vi "FPGA_R_ADC_loadcell_W_DAC.vi"() -> ()   [LabVIEW 2018]
uses:
  <vilib>/rvi/Emulation/niFpgaGetClockAttributes.vi
  <vilib>/rvi/Emulation/niFpgaSctlEmulationGetInTimedLoop.vi
  <vilib>/rvi/Emulation/niFpgaEmulationReportErrorSimple.vi
  <vilib>/rvi/eio/common/nirviEmuTemplateMethod_errors.vi
  <vilib>/rvi/Emulation/niFpgaCriticalErrorInLSC.vi
  <vilib>/eio/EIONode/EIONode.xnode
panel:
  out "Data array":bool[](array[boolean])
  in  "stop":bool
  in  "DAC 3 write":bool[](array[boolean])=[FALSE, FALSE, FALSE, FALSE, FALSE, FALSE, FALSE, FALSE, FALSE, FALSE, FALSE, FALSE, FALSE, FALSE, FALSE, FALSE]
  in  "DAC 2 write":bool[](array[boolean])=[FALSE, FALSE, FALSE, FALSE, FALSE, FALSE, FALSE, FALSE, FALSE, FALSE, FALSE, FALSE, FALSE, FALSE, FALSE, FALSE]
  in  "DAC 1 write":bool[](array[boolean])=[FALSE, FALSE, FALSE, FALSE, FALSE, FALSE, FALSE, FALSE, FALSE, FALSE, FALSE, FALSE, FALSE, FALSE, FALSE, FALSE]
  out "ADC read":bool[](array[boolean])
  in  "ADC write":bool[](array[boolean])=[FALSE, FALSE, FALSE, FALSE, FALSE, TRUE, FALSE, FALSE, FALSE, FALSE, FALSE, FALSE, FALSE, FALSE, FALSE, FALSE]
  in  "Stop":bool
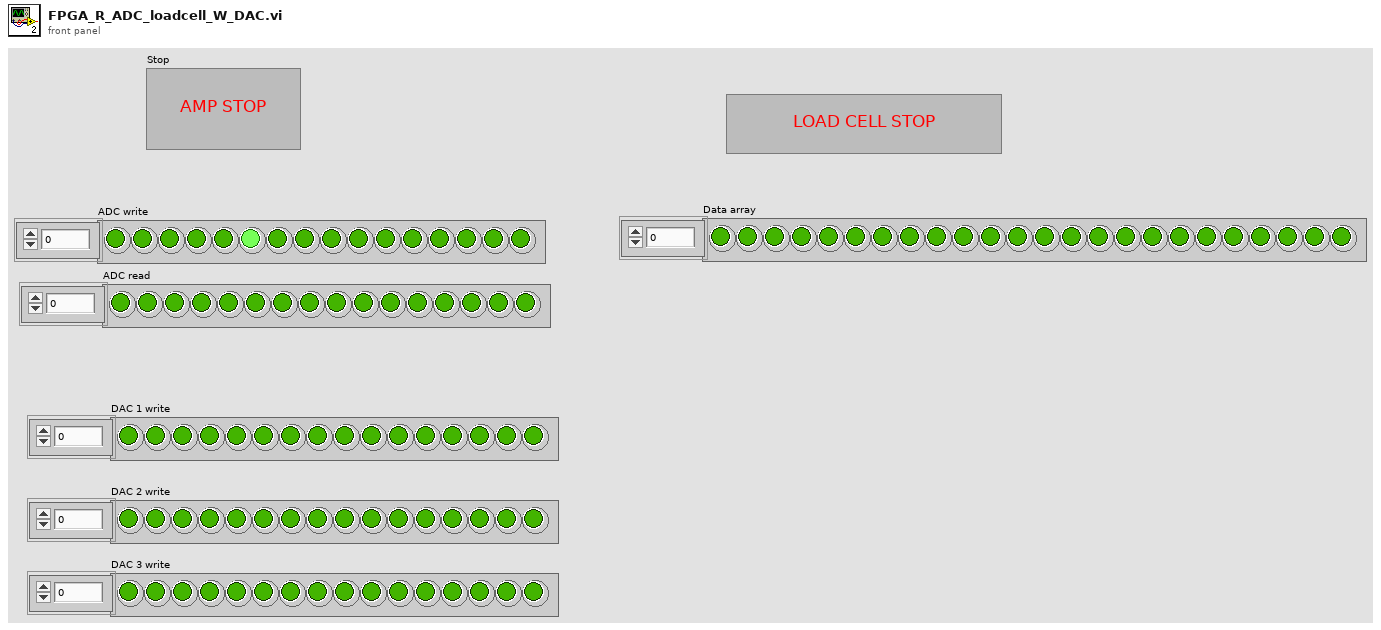
[diagram p1: front panel]
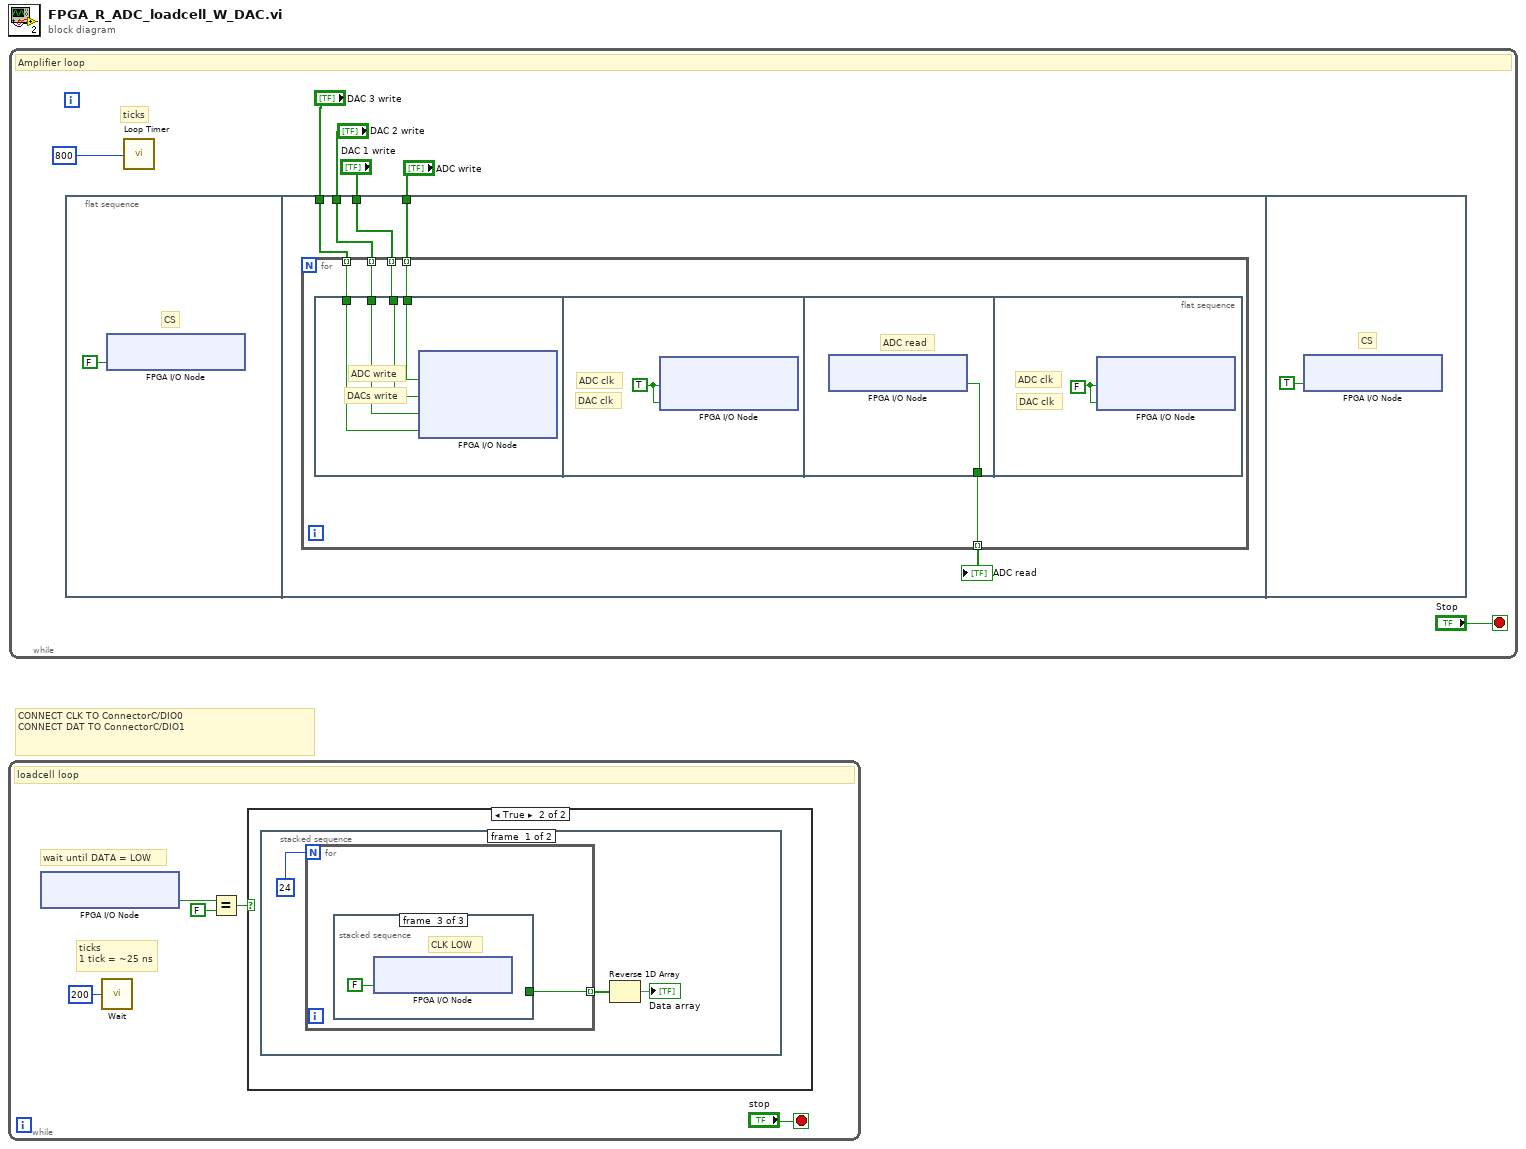
[diagram p0: block diagram]
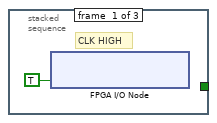
[diagram p3: hidden frame]
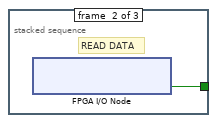
[diagram p4: hidden frame]
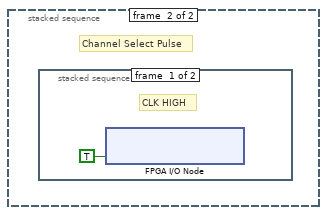
[diagram p5: hidden frame]
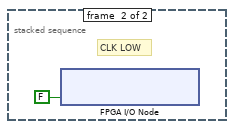
[diagram p6: hidden frame]
diagram:
  # "CONNECT CLK TO ConnectorC/DIO0\nCONNECT DAT TO ConnectorC/DIO1"
  n1 = while {
    stop <- "stop" stop-if-true
    # "ticks\n1 tick = ~25 ns"
    # "wait until DATA = LOW"
    # "loadcell loop"
    n2 = xnode "FPGA I/O Node"() -> ("ConnectorC/DIO1"=w4:bool)  [unwired: 1 in, 1 out]
    n3 = call "Wait"("Count(Ticks)"=u32 200) -> ()  [unwired: 1 out]
    n4 = Equal?(x=w4, y=FALSE) -> (x = y?=w2:bool)
    n5 = case shown="True" w2 {
      frame False {
      }
      frame True {
        n6 = stacked-sequence {
          frame #0 {
            n7 = for {
              N: 24 -> [_]
              tunnel: [w9] -> w7 mode=indexing
              n8 = stacked-sequence {
                tunnel: [_ w11 _] -> w9
                frame #0 {
                  # "CLK HIGH"
                  n9 = xnode "FPGA I/O Node"("ConnectorC/DIO0"=TRUE ("ConnectorB/DIO0")) -> ()  [unwired: 1 in, 1 out]
                }
                frame #1 {
                  # "READ DATA"
                  n10 = xnode "FPGA I/O Node"() -> ("ConnectorC/DIO1"=w11:bool)  [unwired: 1 in, 1 out]
                }
                frame #2 {
                  # "CLK LOW"
                  n11 = xnode "FPGA I/O Node"("ConnectorC/DIO0"=FALSE ("ConnectorB/DIO0")) -> ()  [unwired: 1 in, 1 out]
                }
              }
            }
            n12 = Reverse 1D Array(array=w7) -> (reversed array=→"Data array":bool[])
          }
          frame #1 {
            # "Channel Select Pulse"
            n13 = stacked-sequence {
              frame #0 {
                # "CLK HIGH"
                n14 = xnode "FPGA I/O Node"("ConnectorC/DIO0"=TRUE ("ConnectorB/DIO0")) -> ()  [unwired: 1 in, 1 out]
              }
              frame #1 {
                # "CLK LOW"
                n15 = xnode "FPGA I/O Node"("ConnectorC/DIO0"=FALSE ("ConnectorB/DIO0")) -> ()  [unwired: 1 in, 1 out]
              }
            }
          }
        }
      }
    }
  }
  n16 = while {
    stop <- "Stop" stop-if-true
    # "ticks"
    # "Amplifier loop"
    n17 = flat-sequence {
      tunnel: "ADC write" -> [w26]
      tunnel: "DAC 1 write" -> [w24]
      tunnel: "DAC 2 write" -> [w23]
      tunnel: "DAC 3 write" -> [w22]
      frame #0 {
        # "CS"
        n18 = xnode "FPGA I/O Node"("ConnectorA/DIO4"=FALSE) -> ()  [unwired: 1 in, 1 out]
      }
      frame #1 {
        n19 = for {
          tunnel: w26 -> [w31] mode=indexing
          tunnel: [w30] -> w25 mode=indexing
          tunnel: w24 -> [w29] mode=indexing
          tunnel: w23 -> [w28] mode=indexing
          tunnel: w22 -> [w27] mode=indexing
          n20 = flat-sequence {
            tunnel: w31 -> [w35]
            tunnel: w29 -> [w34]
            tunnel: w28 -> [w33]
            tunnel: w27 -> [w32]
            tunnel: [w37] -> w30
            frame #0 {
              # "DACs write"
              # "ADC write"
              n21 = xnode "FPGA I/O Node"("ConnectorA/DIO2"=w35, "ConnectorA/DIO6"=w34, "ConnectorA/DIO7"=w33, "ConnectorA/DIO8"=w32) -> ()  [unwired: 4 in, 4 out]
            }
            frame #1 {
              w36 = TRUE ("ConnectorA/DIO3")
              # "DAC clk"
              # "ADC clk"
              n22 = xnode "FPGA I/O Node"("ConnectorA/DIO3"=w36, "ConnectorA/DIO5"=w36) -> ()  [unwired: 2 in, 2 out]
            }
            frame #2 {
              # "ADC read"
              n23 = xnode "FPGA I/O Node"() -> ("ConnectorA/DIO1"=w37:bool)  [unwired: 1 in, 1 out]
            }
            frame #3 {
              w38 = FALSE ("ConnectorA/DIO3")
              # "DAC clk"
              # "ADC clk"
              n24 = xnode "FPGA I/O Node"("ConnectorA/DIO3"=w38, "ConnectorA/DIO5"=w38) -> ()  [unwired: 2 in, 2 out]
            }
          }
        }
        "ADC read" <- w25
      }
      frame #2 {
        # "CS"
        n25 = xnode "FPGA I/O Node"("ConnectorA/DIO4"=TRUE) -> ()  [unwired: 1 in, 1 out]
      }
    }
    n26 = call "Loop Timer"("Count(Ticks)"=u32 800) -> ()  [unwired: 1 out]
  }
